vi "Single Mic Test.vi"(0 "Peiker_Stepped Sweep Settings":T3={"Input Settings"={"IEPE min time to settle [s]"=0.0, "Responce Channel Settings"={"DSA response channel settings"={"coupling"=10045, "enable IEPE excitation"=FALSE, "IEPE current [mA]"=4.0}, "response channel info"={"sensor sensitivity"=1000.0, "engineering units"=1, "dB reference"=1.0, "custom label"="EU", "weighting filter"=0, "pregain"=0.0}, "AI response settings"={"response channel"="SOUNDACQ/ai1", "max value [V]"=10.0, "min value [V]"=-10.0, "terminal configuration"=-1}}, "Stimulus Channel Settings"={"AI stimulus settings"={"stimulus channel"="SOUNDACQ/ai0", "max value [V]"=10.0, "min value [V]"=-10.0, "terminal configuration"=-1}, "DSA stimulus channel settings"={"coupling"=10045, "enable IEPE excitation"=TRUE, "IEPE current [mA]"=4.0}, "stimulus channel info"={"sensor sensitivity"=11.4, "engineering units"=2, "dB reference"=2e-05, "custom label"="EU", "weighting filter"=0, "pregain"=0.0}}}, "Output Settings"={"AO source settings"={"excitation channel"="SOUNDACQ/ao0", "max value [V]"=10.0, "min value [V]"=-10.0, "terminal configuration"=-1}}} {"Output Settings"."AO source settings"."terminal configuration" items=["Default"=-1, "RSE"=10083, "Differential"=10106, "Pseudodifferential"=12529]; "Output Settings"."AO source settings"."min value [V]" format="%0.2f"; "Output Settings"."AO source settings"."max value [V]" format="%0.2f"; "Input Settings"."Stimulus Channel Settings"."stimulus channel info"."pregain" format="%.2f"; "Input Settings"."Stimulus Channel Settings"."stimulus channel info"."weighting filter" items=["Linear", "A-weighting", "B-weighting", "C-weighting", "ITU-R 468-4", "Dolby", "CCITT", "C-message", "Wb", "Wc", "Wd", "We", "Wf", "Wh", "Wj", "Wk", "Wm", "AES17 20 kHz lowpass", "AES17 40 kHz lowpass", "AES17 20 kHz highpass", "AES17 40 kHz highpass"]; "Input Settings"."Stimulus Channel Settings"."stimulus channel info"."dB reference" format="%^.1e"; "Input Settings"."Stimulus Channel Settings"."stimulus channel info"."engineering units" items=["custom..."=0, "V"=1, "A"=21, "C"=30, "pC"=31, "s"=32, "-"=29, "Pa"=2, "N"=20, "g"=3, "m/s^2"=4, "m/s"=5, "m"=6, "mm/s"=12, "mm"=13, "micron/s"=14, "micron"=15, "in/s^2"=7, "in/s"=8, "in"=9, "mil/s"=10, "mil"=11, "rad/s^2"=16, "rad/s"=17, "rad"=18, "deg/s^2"=26, "deg/s"=27, "deg"=28, "RPM"=22, "cycle/s^2"=23, "Hz"=24, "cycle"=25, "strain"=19]; "Input Settings"."Stimulus Channel Settings"."stimulus channel info"."sensor sensitivity" format="%#_5f"; "Input Settings"."Stimulus Channel Settings"."DSA stimulus channel settings"."IEPE current [mA]" format="%.1f"; "Input Settings"."Stimulus Channel Settings"."DSA stimulus channel settings"."coupling" items=["AC"=10045, "DC"=10050, "GND"=10066]; "Input Settings"."Stimulus Channel Settings"."AI stimulus settings"."terminal configuration" items=["Default"=-1, "RSE"=10083, "NRSE"=10078, "Differential"=10106, "Pseudodifferential"=12529]; "Input Settings"."Stimulus Channel Settings"."AI stimulus settings"."min value [V]" format="%.2f"; "Input Settings"."Stimulus Channel Settings"."AI stimulus settings"."max value [V]" format="%.2f"; "Input Settings"."Responce Channel Settings"."AI response settings"."terminal configuration" items=["Default"=-1, "RSE"=10083, "NRSE"=10078, "Differential"=10106, "Pseudodifferential"=12529]; "Input Settings"."Responce Channel Settings"."AI response settings"."min value [V]" format="%.2f"; "Input Settings"."Responce Channel Settings"."AI response settings"."max value [V]" format="%.2f"; "Input Settings"."Responce Channel Settings"."response channel info"."pregain" format="%.2f"; "Input Settings"."Responce Channel Settings"."response channel info"."weighting filter" items=["Linear", "A-weighting", "B-weighting", "C-weighting", "ITU-R 468-4", "Dolby", "CCITT", "C-message", "Wb", "Wc", "Wd", "We", "Wf", "Wh", "Wj", "Wk", "Wm", "AES17 20 kHz lowpass", "AES17 40 kHz lowpass", "AES17 20 kHz highpass", "AES17 40 kHz highpass"]; "Input Settings"."Responce Channel Settings"."response channel info"."dB reference" format="%^.1e"; "Input Settings"."Responce Channel Settings"."response channel info"."engineering units" items=["custom..."=0, "V"=1, "A"=21, "C"=30, "pC"=31, "s"=32, "-"=29, "Pa"=2, "N"=20, "g"=3, "m/s^2"=4, "m/s"=5, "m"=6, "mm/s"=12, "mm"=13, "micron/s"=14, "micron"=15, "in/s^2"=7, "in/s"=8, "in"=9, "mil/s"=10, "mil"=11, "rad/s^2"=16, "rad/s"=17, "rad"=18, "deg/s^2"=26, "deg/s"=27, "deg"=28, "RPM"=22, "cycle/s^2"=23, "Hz"=24, "cycle"=25, "strain"=19]; "Input Settings"."Responce Channel Settings"."response channel info"."sensor sensitivity" format="%#_5f"; "Input Settings"."Responce Channel Settings"."DSA response channel settings"."IEPE current [mA]" format="%.1f"; "Input Settings"."Responce Channel Settings"."DSA response channel settings"."coupling" items=["AC"=10045, "DC"=10050, "GND"=10066]; "Input Settings"."IEPE min time to settle [s]" format="%.1f"}, 1 "Freq Response Limit":cluster{"Freq":dbl, "Upper":dbl, "Lower":dbl}[](array[cluster]), 5 "frequency list Input":T8(array[cluster])=[{"frequency [Hz]"=103.0, "amplitude [V]"=0.09342446715491094}] {"amplitude [V]" format="%.6f"; "frequency [Hz]" format="%.2f"}, 7 "Error In":errorcluster, 9 "Test Level":T2={"FrequencyList Input Level (dBSPL)"=94.0, "FrequencyList Output Level (dBSPL) 2"=94.0}, 11 "Model (T-79)":bool, 12 "dB Reference":dbl=84.0, 14 "String":string) -> (4 "ProcessedFrequencyResponse":dbl[](array[numeric]), 6 "Processed Freq Response":T1(graph) caption="Fundamental-Response Mic1", 10 "Test Result Out":dbl[](array[numeric]), 15 "Error Out":errorcluster)   [LabVIEW 2018]
uses:
  Microfontest/Peiker_Stepped Sweep Settings.ctl
  <vilib>/addons/_NISVFA/_Shared subVIs/Controls/svc_DSA Channel Settings.ctl
  <vilib>/addons/_NISVFA/_Shared subVIs/Controls/svc_Channel Info.ctl
  <vilib>/addons/_NISVFA/_Shared subVIs/Controls/svc_Engineering Units Text Ring.ctl
  <vilib>/addons/_NISVFA/_Shared subVIs/Controls/svc_Weighting Filter Text Ring.ctl
panel:
  # "Single Mic Test"
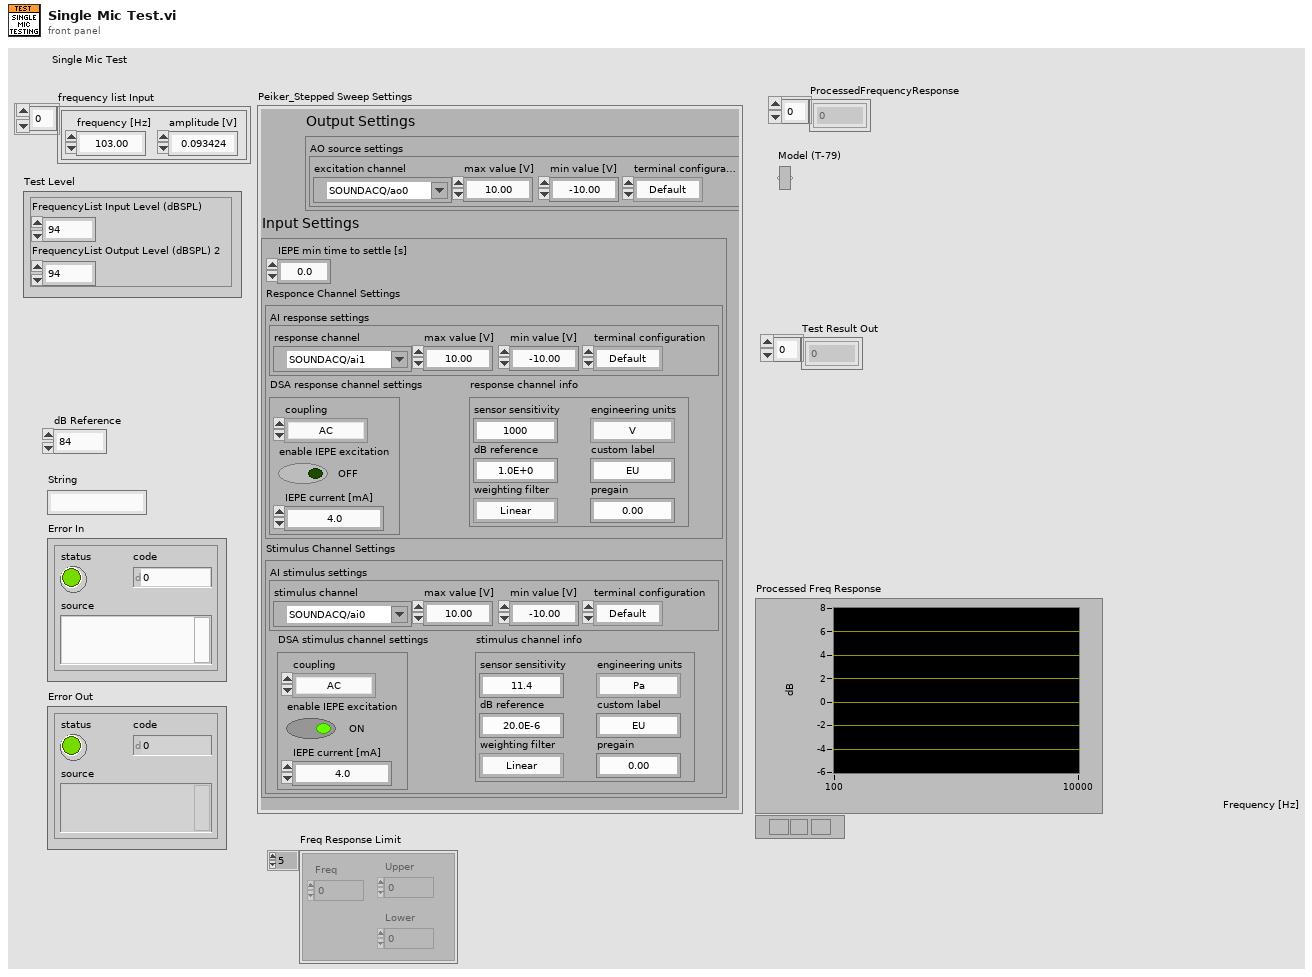
[diagram p1: front panel]
types:
  T1 = cluster{"frequency [Hz]":dbl[], "amplitude":dbl[]}
  T2 = cluster{"FrequencyList Input Level (dBSPL)":dbl, "FrequencyList Output Level (dBSPL) 2":dbl}
  T3 = typedef "Peiker_Stepped Sweep Settings.ctl" = cluster{"Input Settings":cluster{"IEPE min time to settle [s]":dbl, "Responce Channel Settings":cluster{"DSA response channel settings":T4, "response channel info":T5, "AI response settings":cluster{"response channel":tag, "max value [V]":dbl, "min value [V]":dbl, "terminal configuration":i32}}, "Stimulus Channel Settings":cluster{"AI stimulus settings":cluster{"stimulus channel":tag, "max value [V]":dbl, "min value [V]":dbl, "terminal configuration":i32}, "DSA stimulus channel settings":T4, "stimulus channel info":T5}}, "Output Settings":cluster{"AO source settings":cluster{"excitation channel":tag, "max value [V]":dbl, "min value [V]":dbl, "terminal configuration":i32}}}
  T4 = typedef "svc_DSA Channel Settings.ctl" = cluster{"coupling":i32, "enable IEPE excitation":bool, "IEPE current [mA]":dbl}
  T5 = typedef "svc_Channel Info.ctl" = cluster{"sensor sensitivity":dbl, "engineering units":T6, "dB reference":dbl, "custom label":string, "weighting filter":T7, "pregain":dbl}
  T6 = typedef "svc_Engineering Units Text Ring.ctl" = u16
  T7 = typedef "svc_Weighting Filter Text Ring.ctl" = u16
  T8 = cluster{"frequency [Hz]":dbl, "amplitude [V]":dbl}[]
  T9 = cluster{"settle time [s]":dbl, "settle cycles":i32}
  T10 = cluster{"integration time [s]":dbl, "integration cycles":i32}
  T11 = cluster{"frequency [Hz]":dbl, "amplitude [V]":dbl}
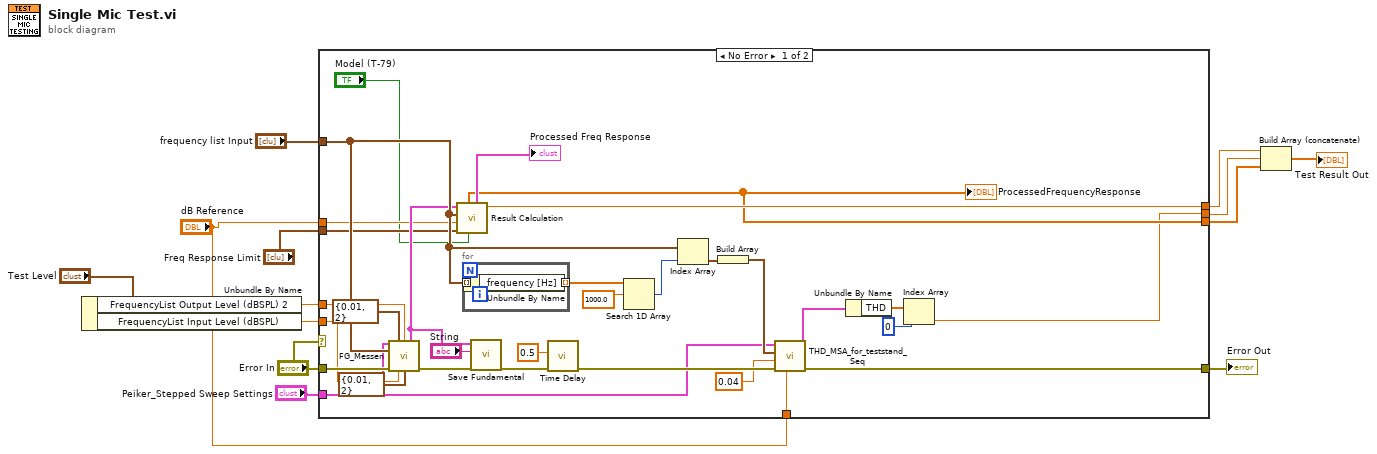
[diagram p0: block diagram]
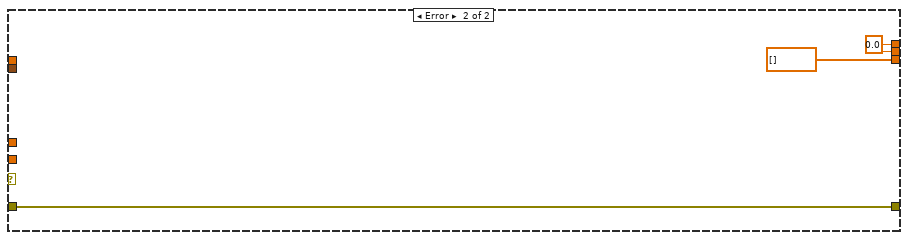
[diagram p2: hidden frame]
diagram:
  n1 = Unbundle By Name("Test Level") -> ("FrequencyList Output Level (dBSPL) 2"=w8:dbl, "FrequencyList Input Level (dBSPL)"=w7:dbl)
  n2 = case shown="No Error" "Error In" {
    tunnel: "Error In" -> [w44 w49]
    tunnel: "frequency list Input" -> [w39 _]
    tunnel: "Peiker_Stepped Sweep Settings" -> [w34 _]
    tunnel: [w32 w49] -> w10
    tunnel: [w31 w47] -> w6
    tunnel: [w28 w47] -> w5
    tunnel: [w30 dbl[] [] ("ProcessedFrequencyResponse")] -> w4
    tunnel: w8 -> [w26 _]
    tunnel: w7 -> [w25 _]
    tunnel: "dB Reference" -> [w20 _]
    tunnel: "dB Reference" -> [w19 _]
    tunnel: "Freq Response Limit" -> [w18 _]
    frame No Error {
      n3 = call "FG_Messen.vi"("Peiker_Stepped Sweep Settings"=w34, "settling time"=T9 {"settle time [s]"=0.01, "settle cycles"=2}, "FrequencyList Output Level (dBSPL)"=w26, "frequency list Input"=w39, "error in (no error)"=w44, "FrequencyList Input Level (dBSPL)"=w25, "integration time"=T10 {"integration time [s]"=0.01, "integration cycles"=2}) -> ("Fundamental-Response"=w22:T1, "error out"=w24:errorcluster)  [unwired: 2 in, 5 out]
      n4 = call "Result Calculation.vi"("shifting"="Model (T-79)", "Freq Response Limit"=w18, "dB Reference"=w20, "Frequency List"=w39, "Fundamental-Response"=w22) -> ("Sensitivity (dBSPL)"=w31:dbl, "Processed Freq Response"=→"Processed Freq Response":T1, "ProcessedFrequencyResponse"=w30:dbl[])  [unwired: 3 in, 1 out]
      "ProcessedFrequencyResponse" <- w30
      n5 = for {
        tunnel: w39 -> [w46] mode=indexing
        tunnel: [w45] -> w38 mode=indexing
        n6 = Unbundle By Name(w46) -> ("frequency [Hz]"=w45:dbl)
      }
      n7 = call "Save Fundamental.vi"("error in (no error)"=w24, "String"="String", "Fundamental-Response"=w22) -> ("error out"=w23:errorcluster)  [unwired: 8 in]
      n8 = call "Time Delay"("error in (no error)"=w23, "Delay Time (s)"=0.5) -> ("error out"=w41:errorcluster)  [unwired: 9 in]
      n9 = Search 1D Array(1D array=w38, element=1000.0 ("index")) -> (index of element=w37:i32)  [unwired: 1 in]
      n10 = Index Array(array=w39, index=w37) -> (element=w36:T11)
      n11 = Build Array(w36) -> (w35:T8)
      n12 = call "THD_MSA_for_teststand_Seq.vi"("Sound_Pressure(dB SPL)"=w19, "error in"=w41, "Std_Deviation_Thresold"=0.04, "frequency list Input"=w35, "Peiker_Stepped Sweep Settings"=w34) -> ("error out"=w32:errorcluster, "THD-Response"=w33:cluster{"frequency":dbl[], "THD":dbl[]})  [unwired: 4 in, 1 out]
      n13 = Unbundle By Name(w33) -> ("THD"=w29:dbl[])
      n14 = Index Array(array=w29, index=0) -> (element=w28:dbl)
    }
    frame Error {
      w47 = 0.0 ("Sensitivity (dBSPL)")
    }
  }
  "Error Out" <- w10
  n15 = Build Array (concatenate)(w6, w5, w4) -> (→"Test Result Out":dbl[])
